vi "test_CloseSink_APICallsDone_SinkDestroyed.vi"(8 "error in (no error)":errorcluster, 11 "TestCase in":refnum<class "TestDataSink.lvclass">) -> (0 "error out":errorcluster, 3 "TestCase out":refnum<class "TestDataSink.lvclass">)   [LabVIEW 2017, in "TestDataSink.lvclass"]
uses:
  TestDataSink.lvclass
  Source/Composed Log/Types/Log Level.ctl
  Source/LVQueue Sink/LVQueue Sink.lvclass/LVQueue Sink.ctl
  Source/Composed Log/LoggerReference/LoggerReference.lvclass/LoggerReference.ctl
  8df0e21b-ffec-424d-9666-e5fc056b1b69.vi
  8df0e21b-ffec-424d-9666-e5fc056b1b69.vi/949d7edf-f65e-4bb7-a5b6-26ad9c933643.vi
  Source/Composed Log/LoggerReference/Return Aggregate Queues.vi
  Source/Composed Log/LoggerReference/Add Aggregate Log.vi
  8df0e21b-ffec-424d-9666-e5fc056b1b69.vi/949d7edf-f65e-4bb7-a5b6-26ad9c933643.vi/ba470c74-13db-4926-8fca-c726079f5153.vi
  Source/Composed Log/LoggerReference/Send Add Sink.vi
  Source/LVQueue Sink/LVQueue Sink.lvclass
  C:/CS/Internal/LabVIEW/Logger/Source/Composed Log/Log Sink/Log Sink.lvclass
  Source/Composed Log/Application Logger/Launch Worker Loop.vi
  Source/Composed Log/LoggerReference/Initialize Logger Instance.vi
  Source/Composed Log/Singleton Event Log/Logger Queue FGV.vi
  Source/Composed Log/IErrorFormat/IErrorFormat.lvclass
  Source/Composed Log/LoggerReference/LoggerReference.lvclass
  Source/Composed Log/Log Sink/Log Sink.lvclass
  Source/Composed Log/Singleton Event Log/Singleton Event Log.lvlib
  Source/Composed Log/Composed Log.lvlib
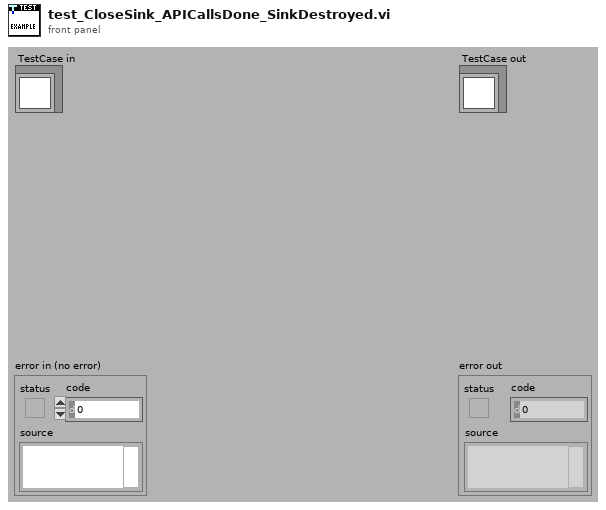
[diagram p1: front panel]
types:
  T1 = typedef "Composed Log.lvlib/Log Level.ctl" = enum16{"Debug", "Info", "Warning", "Error", "Critical"}
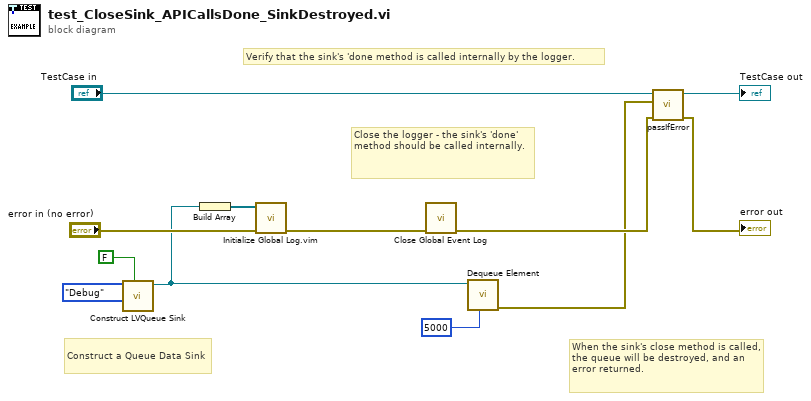
[diagram p0: block diagram]
diagram:
  # "Verify that the sink's 'done method is called internally by the logger."
  # "When the sink's close method is called, the queue will be destroyed, and an error returned."
  # "Close the logger - the sink's 'done' method should be called internally."
  # "Construct a Queue Data Sink"
  n1 = call "Construct LVQueue Sink.vi"("User Shutdown? (F)"=FALSE, "LogLevel"=Log_Level."Debug") -> ("LVQueue Sink out"=w8:refnum<class "LVQueue Sink.lvclass">)  [unwired: 8 in, 1 out]
  n2 = Build Array(w8) -> (w7:refnum<class "LVQueue Sink.lvclass">[])
  n3 = call "Initialize Global Log.vim"("error in (no error)"="error in (no error)", "Log Sink(s)"=w7) -> ("error out"=w3:errorcluster)  [unwired: 8 in, 1 out]
  n4 = call "Close Global Event Log.vi"("error in (no error)"=w3) -> ("error out"=w4:errorcluster)  [unwired: 10 in]
  n5 = call "Dequeue Element.vi"("timeout in ms (-1)"=5000, "LVQueue Sink in"=w8) -> ("error out"=w2:errorcluster)  [unwired: 6 in, 3 out]
  n6 = call-dynamic "passIfError.vi"("error in (no error)"=w4, "error"=w2, "TestCase in"="TestCase in") -> ("error out"=→"error out":errorcluster, "TestCase out"=→"TestCase out":refnum<class "TestDataSink.lvclass">)  [unwired: 7 in]
